vi "Read Log Path.vi"(7 "key":string, 8 "error in (no error)":errorcluster, 10 "refnum":T1, 11 "Process in":refnum<class "Process.lvclass">) -> (0 "error out":errorcluster, 1 "value":path, 2 "refnum out":T1, 3 "Process out":refnum<class "Process.lvclass">)   [LabVIEW 2020, in "Configuration File.lvlib"]
doc: "High-level function for reading configuration file data from process class."
uses:
  Configuration File.lvlib
  Process Classes/Process/Process.lvclass
  <vilib>/Utility/config.llb/Config Data RefNum.ctl
  <vilib>/Utility/config.llb/Read Key (Path).vi
  <vilib>/Utility/config.llb/Write Key (Path).vi
  <vilib>/Utility/config.llb/NI_LVConfig.lvlib
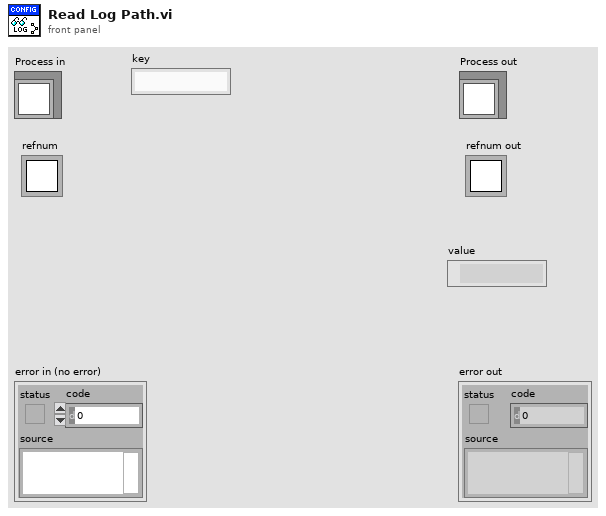
[diagram p1: front panel]
types:
  T1 = typedef "NI_LVConfig.lvlib/Config Data RefNum.ctl" = refnum<k1>
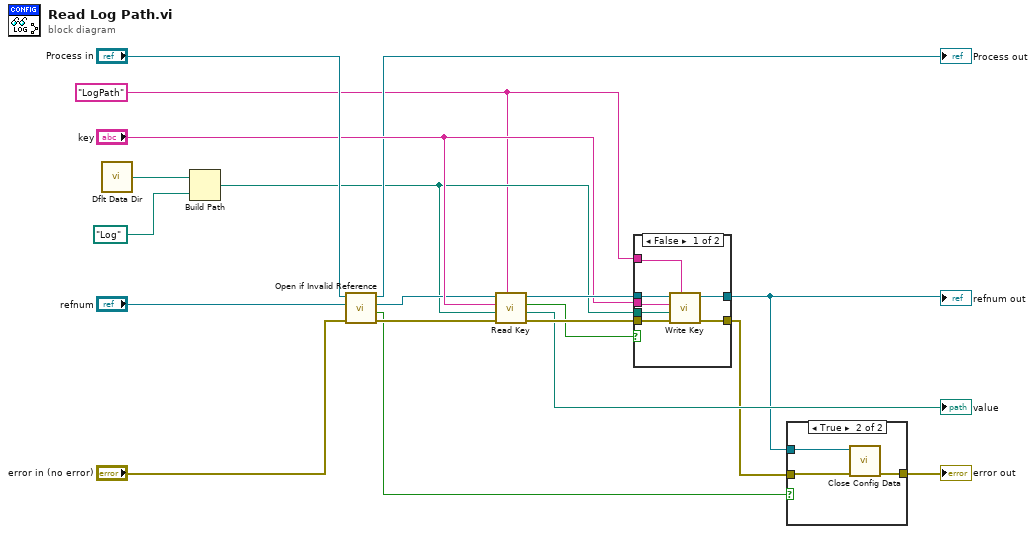
[diagram p0: block diagram]
diagram:
  w1 = "LogPath" ("Process Name")
  n1 = call <vilib>:"Dflt Data Dir.vi"() -> ("App:Default Data Directory"=w2:path)
  n2 = Build Path(base path=w2, name or relative path=path "Log" ("default value")) -> (appended path=w3:path)
  n3 = call "Open if Invalid Reference.vi"("error in (no error)"="error in (no error)", "refnum"="refnum", "Process in"="Process in") -> ("error out"=w10:errorcluster, "File opened?"=w4:bool, "refnum out"=w11:T1, "Process out"=→"Process out":refnum<class "Process.lvclass">)  [unwired: 5 in]
  n4 = call-poly <vilib>:"Read Key.vi"("section"=w1, "error in (no error)"=w10, "default value"=w3, "key"="key", "refnum"=w11) -> ("error out"=w17:errorcluster, "value"=→"value":path, "found?"=w16:bool, "refnum out"=w18:T1)  [unwired: 3 in]
  n5 = case shown="False" w16 {
    tunnel: w18 -> [w26 w28]
    tunnel: w17 -> [w25 w27]
    tunnel: [w24 w28] -> w7
    tunnel: [w23 w27] -> w6
    tunnel: "key" -> [w22 _]
    tunnel: w1 -> [w21 _]
    tunnel: w3 -> [w20 _]
    frame False {
      n6 = call-poly <vilib>:"Write Key.vi"("section"=w21, "error in (no error)"=w25, "value"=w20, "key"=w22, "refnum"=w26) -> ("error out"=w23:errorcluster, "refnum out"=w24:T1)  [unwired: 4 in, 1 out]
    }
    frame True {
    }
  }
  "refnum out" <- w7
  n7 = case shown="True" w4 {
    tunnel: w7 -> [_ w32]
    tunnel: w6 -> [w29 w31]
    tunnel: [w29 w30] -> w5
    frame False {
    }
    frame True {
      n8 = call <vilib>:"Close Config Data.vi"("error in (no error)"=w31, "refnum"=w32) -> ("error out"=w30:errorcluster)  [unwired: 8 in, 1 out]
    }
  }
  "error out" <- w5
